vi "Resistance Test_byDMM_ver2.vi"(0 "DMM ref in":refnum<visa-resource-name>, 2 "Resistance Test REF":refnum<vi>, 3 "Resistance Test Stop REF":refnum<vi>, 5 "DMM error in":errorcluster, 7 "Channel  Count":i32, 9 "ESP32 ref in":refnum<visa-resource-name>="COM4", 11 "ESP32 error in":errorcluster) -> (10 "ESP32 ref out":refnum<visa-resource-name>, 15 "ESP32 error out":errorcluster)   [LabVIEW 2023]
uses:
  <instrlib>/Agilent 3446X Series/Agilent 3446X Series.lvlib
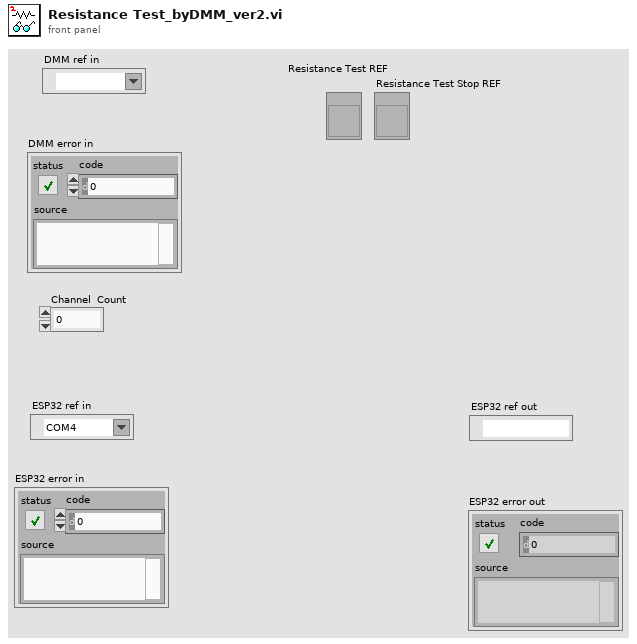
[diagram p1: front panel]
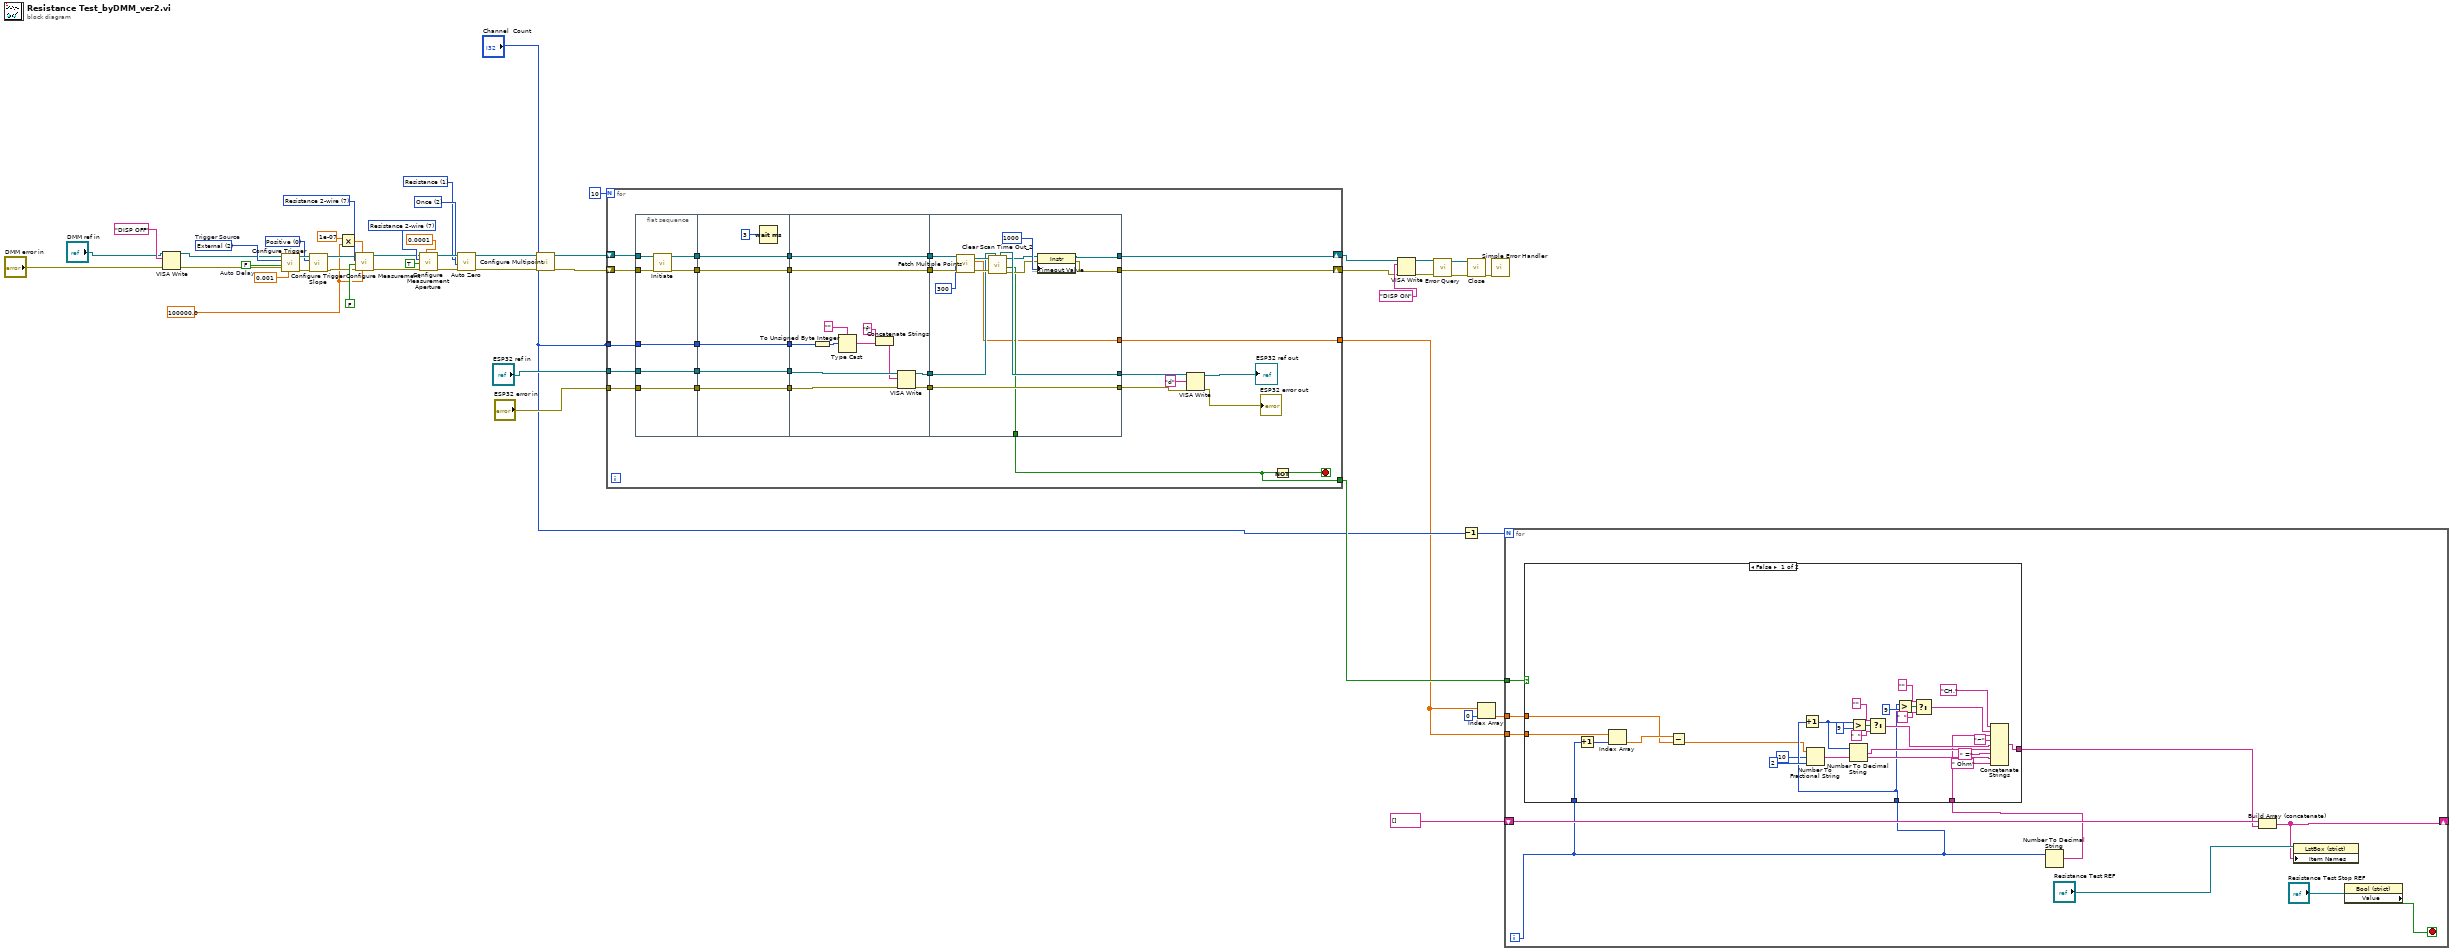
[diagram p0: block diagram]
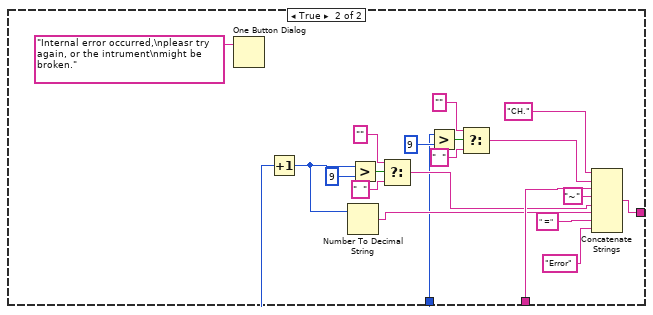
[diagram p2: hidden frame]
diagram:
  w18 = 100000.0 ("Measure\nMax Voltage")
  w31 = 0 items=["Positive", "Negative"] ("Trigger Edge (1: Negative)")
  w29 = 2 items=["Immediate", "Software (Bus)", "External"]  # Trigger Source
  w30 = FALSE  # Auto Delay
  w37 = 7 items=["Continuity", "Current AC", "Current DC", "Diode", "Frequency", "Resistance 4-wire", "Period", "Resistance 2-wire", "Temperature", "Voltage AC", "Voltage DC", "Voltage DC Ratio", "Capacitance"] ("Measurement Function (10: Voltage DC)")
  w43 = 1 items=["Current DC", "Resistance", "Temperature", "Voltage DC"] ("Zero Type (0: Current DC)")
  w44 = 2 items=["Disable", "Enable", "Once"] ("Auto Zero (1: Enable)")
  w40 = 7 items=["Continuity", "Current AC", "Current DC", "Diode", "Frequency", "Resistance 4-wire", "Period", "Resistance 2-wire", "Temperature", "Voltage AC", "Voltage DC", "Voltage DC Ratio", "Capacitance"] ("Measurement Function (0: Continuity)")
  n1 = VISA Write(VISA resource name="DMM ref in", write buffer="DISP OFF", error in (no error)="DMM error in") -> (VISA resource name out=w20:refnum<visa-resource-name>, error out=w19:errorcluster)  [unwired: 1 out]
  n2 = call <instrlib>:"Configure Trigger.vi"("Manual Trigger Delay (1 s)"=0.001, "error in (no error)"=w19, "Auto Delay (F:Disable)"=w30, "Trigger Source (0: Immediate)"=w29, "VISA resource name"=w20) -> ("error out"=w33:errorcluster, "VISA resource name out"=w32:refnum<visa-resource-name>)  [unwired: 1 in, 4 out]
  n3 = call <instrlib>:"Configure Trigger Slope.vi"("error in (no error)"=w33, "Trigger Edge (1: Negative)"=w31, "VISA resource name"=w32) -> ("error out"=w26:errorcluster, "VISA resource name out"=w27:refnum<visa-resource-name>)  [unwired: 7 in]
  n4 = Multiply(x=1e-07, y=w18) -> (x*y=w38:dbl)
  n5 = call <instrlib>:"Configure Measurement.vi"("Manual Range (1)"=w18, "Absolute Resolution (1E-6)"=w38, "error in (no error)"=w26, "Auto Range (T: Enable)"=FALSE, "Measurement Function (10: Voltage DC)"=w37, "VISA resource name"=w27) -> ("error out"=w34:errorcluster, "VISA resource name out"=w35:refnum<visa-resource-name>)  [unwired: 4 out]
  n6 = call <instrlib>:"Configure Measurement Aperture.vi"("Aperture Time (0.1s)"=0.0001, "error in (no error)"=w34, "Enable Aperture (F: Disable)"=TRUE, "Measurement Function (0: Continuity)"=w40, "VISA resource name"=w35) -> ("error out"=w46:errorcluster, "VISA resource name out"=w45:refnum<visa-resource-name>)  [unwired: 5 in]
  n7 = call <instrlib>:"Auto Zero.vi"("error in (no error)"=w46, "Auto Zero (1: Enable)"=w44, "Zero Type (0: Current DC)"=w43, "VISA resource name"=w45) -> ("error out"=w16:errorcluster, "VISA resource name out"=w17:refnum<visa-resource-name>)  [unwired: 6 in]
  n8 = call <instrlib>:"Configure Multipoint.vi"("error in (no error)"=w16, "Trigger Count (1)"="Channel  Count", "VISA resource name"=w17) -> ("error out"=w24:errorcluster, "VISA resource name out"=w25:refnum<visa-resource-name>)  [unwired: 4 in, 3 out]
  n9 = for {
    N: 10 -> [_]
    tunnel: "ESP32 ref in" -> [w65]
    tunnel: "ESP32 error in" -> [w64]
    tunnel: [w56] -> w14
    tunnel: [w55] -> w4
    tunnel: "Channel  Count" -> [_]
    tunnel: "Channel  Count" -> [w52]
    shift-right: [w51] -> w7
    shift-left: w25 -> [w60]
    shift-right: [w50] -> w6
    shift-left: w24 -> [w59]
    stop <- w57 stop-if-true
    n10 = flat-sequence {
      tunnel: w59 -> [w83]
      tunnel: w60 -> [w85]
      tunnel: [w84] -> w78
      tunnel: [w82] -> w77
      tunnel: [w81] -> w76
      tunnel: w65 -> [w81]
      tunnel: w64 -> [w80]
      tunnel: [w80] -> w75
      tunnel: w52 -> [w79]
      tunnel: [w79] -> w54
      tunnel: [w91] -> w71
      tunnel: [w90] -> w72
      tunnel: w78 -> [w91]
      tunnel: w77 -> [w90]
      tunnel: w76 -> [w88]
      tunnel: [w88] -> w73
      tunnel: w75 -> [w87]
      tunnel: [w87] -> w74
      tunnel: w54 -> [w86]
      tunnel: [w86] -> w53
      tunnel: [w103] -> w70
      tunnel: [w102] -> w69
      tunnel: [w101] -> w68
      tunnel: [w100] -> w67
      tunnel: w74 -> [w98]
      tunnel: w73 -> [w99]
      tunnel: w72 -> [w103]
      tunnel: w71 -> [w102]
      tunnel: w53 -> [w92]
      tunnel: [w106] -> w50
      tunnel: [w107] -> w51
      tunnel: w70 -> [w118]
      tunnel: w69 -> [w117]
      tunnel: [w111] -> w61
      tunnel: w68 -> [w112]
      tunnel: [w115] -> w58
      tunnel: w67 -> [w115]
      tunnel: [w105] -> w56
      tunnel: [w104] -> w55
      frame #0 {
        n11 = call <instrlib>:"Initiate.vi"("error in (no error)"=w83, "VISA resource name"=w85) -> ("error out"=w82:errorcluster, "VISA resource name out"=w84:refnum<visa-resource-name>)  [unwired: 8 out]
      }
      frame #1 {
        n12 = Wait (ms)(milliseconds to wait=u32 3) -> ()  [unwired: 1 out]
      }
      frame #2 {
        n13 = To Unsigned Byte Integer(number=w92) -> (unsigned 8bit integer=w95:u8)
        n14 = Type Cast(type="" ("string"), x=w95) -> (*(type *) &x=w94:string)
        n15 = Concatenate Strings("f" ("data in"), w94) -> (w93:string)
        n16 = VISA Write(VISA resource name=w99, write buffer=w93, error in (no error)=w98) -> (VISA resource name out=w101:refnum<visa-resource-name>, error out=w100:errorcluster)  [unwired: 1 out]
      }
      frame #3 {
        n17 = call <instrlib>:"Fetch Multiple Points.vi"("error in (no error)"=w118, "Timeout (10000 ms)"=300, "VISA resource name"=w117) -> ("error out"=w113:errorcluster, "Measurements"=w104:dbl[], "VISA resource name out"=w114:refnum<visa-resource-name>)  [unwired: 1 in, 5 out]
        n18 = call "Clear Scan Time Out_2.vi"("ESP32 ref"=w112, "error in (no error)"=w113, "VISA Refnum in"=w114) -> ("error out"=w108:errorcluster, "error?"=w105:bool, "VISA Refnum out"=w109:refnum<visa-resource-name>, "ESP32 ref out"=w111:refnum<visa-resource-name>)  [unwired: 4 in, 1 out]
        n19 = property class="Instr"(reference=w109, error in=w108, "General Settings:Timeout Value"=u32 1000) -> (reference out=w107:refnum<visa-resource-name>, error out=w106:errorcluster)
      }
    }
    n20 = VISA Write(VISA resource name=w61, write buffer="d" ("data in"), error in (no error)=w58) -> (VISA resource name out=→"ESP32 ref out":refnum<visa-resource-name>, error out=→"ESP32 error out":errorcluster)  [unwired: 1 out]
    n21 = Not(x=w56) -> (.not. x?=w57:bool)
  }
  n22 = VISA Write(VISA resource name=w7, write buffer="DISP ON", error in (no error)=w6) -> (VISA resource name out=w12:refnum<visa-resource-name>, error out=w13:errorcluster)  [unwired: 1 out]
  n23 = call <instrlib>:"Error Query.vi"("error in (no error)"=w13, "VISA resource name"=w12) -> ("error out"=w9:errorcluster, "VISA resource name out"=w10:refnum<visa-resource-name>)  [unwired: 8 out]
  n24 = Decrement(x="Channel  Count") -> (x-1=w1:i32)
  n25 = call <instrlib>:"Close.vi"("error in (no error)"=w9, "VISA resource name"=w10) -> ("error out"=w11:errorcluster)  [unwired: 9 out]
  n26 = Index Array(array=w4, index=0) -> (element=w2:dbl)
  n27 = call <vilib>:"Simple Error Handler.vi"("error in (no error)"=w11) -> ()  [unwired: 1 in, 8 out]
  n28 = for {
    N: w1 -> [_]
    tunnel: w14 -> [w124]
    shift-right: [w123] -> _
    shift-left: string[] [] -> [w129]
    tunnel: w4 -> [w121]
    tunnel: w2 -> [w119]
    i -> [w120]
    stop <- w122 stop-if-true
    n29 = Number To Decimal String(number=w120) -> (decimal integer string=w125:string)  [unwired: 1 in]
    n30 = case shown="False" w124 {
      tunnel: [w152 w172] -> w127
      tunnel: w125 -> [w137 w169]
      tunnel: w120 -> [w138 w160]
      tunnel: w121 -> [w135 _]
      tunnel: w120 -> [w134 _]
      tunnel: w119 -> [w130 _]
      frame False {
        n31 = Increment(x=w134) -> (x+1=w133:i32)
        n32 = Index Array(array=w135, index=w133) -> (element=w131:dbl)
        n33 = Subtract(x=w131, y=w130) -> (x-y=w132:dbl)
        n34 = Increment(x=w138) -> (x+1=w143:i32)
        n35 = Number To Fractional String(number=w132, width (-)=i16 10, precision (6)=i16 2) -> (F-format string=w140:string)  [unwired: 1 in]
        n36 = Number To Decimal String(number=w143) -> (decimal integer string=w142:string)  [unwired: 1 in]
        n37 = Greater?(x=w143, y=9) -> (0:w147:bool)
        n38 = Select(t="" ("string"), s=w147, f="  " ("string")) -> (s? t:f=w144:string)
        n39 = Greater?(x=w138, y=9) -> (0:w155:bool)
        n40 = Select(t="" ("string"), s=w155, f="  " ("string")) -> (s? t:f=w150:string)
        n41 = Concatenate Strings("CH." ("string"), w150, w137, "~" ("string"), w144, w142, " =" ("string"), w140, " Ohm" ("string")) -> (w152:string)
      }
      frame True {
        n42 = One Button Dialog(message="Internal error occurred,\npleasr try again, or the intrument\nmight be broken.") -> ()  [unwired: 1 in, 1 out]
        n43 = Increment(x=w160) -> (x+1=w162:i32)
        n44 = Number To Decimal String(number=w162) -> (decimal integer string=w161:string)  [unwired: 1 in]
        n45 = Greater?(x=w162, y=9) -> (0:w166:bool)
        n46 = Select(t="" ("string"), s=w166, f="  " ("string")) -> (s? t:f=w163:string)
        n47 = Greater?(x=w160, y=9) -> (0:w175:bool)
        n48 = Select(t="" ("string"), s=w175, f="  " ("string")) -> (s? t:f=w170:string)
        n49 = Concatenate Strings("CH." ("string"), w170, w169, "~" ("string"), w163, w161, " =" ("string"), "Error" ("string")) -> (w172:string)
      }
    }
    n50 = Build Array (concatenate)(w129, w127) -> (w123:string[])
    n51 = property class="LstBox (strict)"(reference="Resistance Test REF", "Item Names"=w123) -> ()  [unwired: 1 in, 2 out]
    n52 = property class="Bool (strict)"(reference="Resistance Test Stop REF") -> ("Value"=w122:bool)  [unwired: 1 in, 2 out]
  }
